vi "get-new-can-frame-by-tag.vi"(8 "error in (no error)":errorcluster, 10 "tag":string, 11 "CANtable in":refnum<class "bAPPdata.lvclass">) -> (0 "error out":errorcluster, 1 "CAN frame":T2 {"payload" format="%x"; "timestamp" format="%<%.7X\n%x>T"; "type" items=["CAN Data"=0, "CAN Remote"=1, "CAN Bus Error"=2, "J1939 Data"=192, "Delay"=224, "Log Trigger"=225, "Start Trigger"=226]; "identifier" format="%x"}, 3 "CANtable out":refnum<class "bAPPdata.lvclass">, 4 "frame.type":T1)   [LabVIEW 2015, in "bAPPdata.lvclass"]
uses:
  bAPPdata.lvclass
  <vilib>/xnet/xnet.llb/XNET Frame CAN.ctl
  <vilib>/xnet/xnet.llb/XNET Frame Type CAN.ctl
  subs/frame.type.ctl
  bAPPdata.lvclass/bAPPdata.ctl
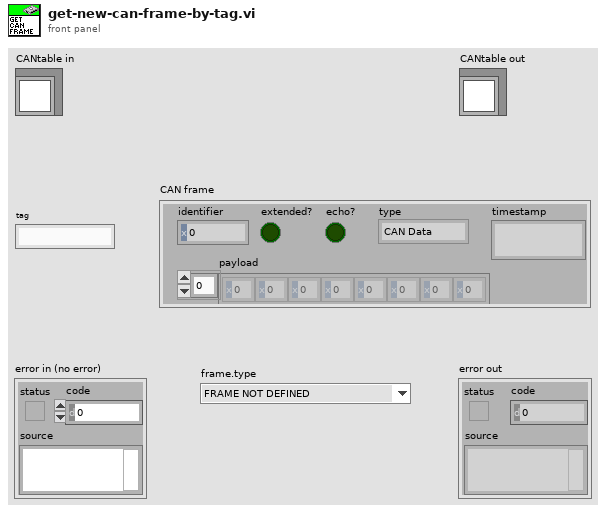
[diagram p1: front panel]
types:
  T1 = typedef "frame.type.ctl" = enum16{"FRAME NOT DEFINED", "DUT OUTPUT FRAME", "DUT INPUT FRAME"}
  T2 = typedef "XNET Frame CAN.ctl" = cluster{"timestamp":timestamp, "payload":u8[], "identifier":u32, "type":T3, "extended?":bool, "echo?":bool}
  T3 = typedef "XNET Frame Type CAN.ctl" = u8
  T4 = typedef "bAPPdata.lvclass/table-data.ctl" = T5[]
  T5 = typedef "bAPPdata.lvclass/table-contents.ctl" = cluster{"id":u32, "tag":string, "frame.type":T1, "last.frame":T2, "tMsgData":T6, "child.tags":string[], "bit-payload":bool[]}
  T6 = typedef "nMsgData.ctl" = cluster{"dwID":u32, "count":u32, "dwCycleTime":dbl, "dwTime":dbl, "new msg":bool}
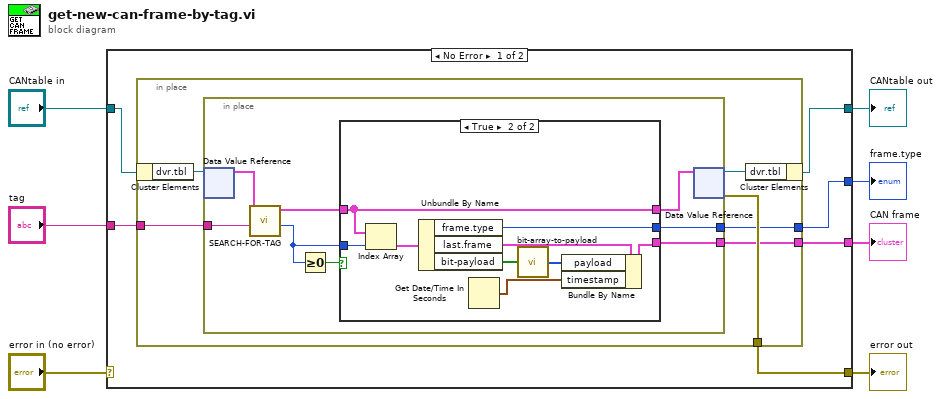
[diagram p0: block diagram]
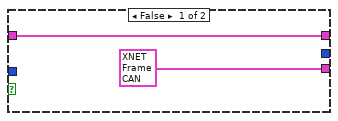
[diagram p2: hidden frame]
diagram:
  n1 = case shown="No Error" "error in (no error)" {
    selector: "error in (no error)" -> [_ w40]
    tunnel: [w8 w40] -> w6
    tunnel: [w12 w39] -> w4
    tunnel: "CANtable in" -> [w13 w39]
    tunnel: "tag" -> [w11 _]
    tunnel: [w10 _] -> w2
    tunnel: [w9 _] -> w1
    frame No Error {
      n2 = in-place {
        in-place-border: w11 -> [w16]
        in-place-border: [w15] -> w10
        in-place-border: [w14] -> w9
        in-place-border: [w19] -> w8
        n3 = in-place-cluster #1(w13) -> ("dvr.tbl"=w18:refnum<data-value>)
        n4 = in-place {
          in-place-border: w16 -> [w26]
          in-place-border: [w22] -> w15
          in-place-border: [w20] -> w14
          n5 = in-place-dvr #2(w18) -> (w27:T4)  [unwired: 1 out]
          n6 = call "SEARCH-FOR-TAG.vi"("tag"=w26, "tbl.list"=w27) -> ("idx"=w21:i32, "tbl.list out"=w24:T5[])  [unwired: 8 in]
          n7 = Greater Or Equal To 0?(x=w21) -> (x >= 0?=w25:bool)
          n8 = case shown="True" w25 {
            tunnel: w24 -> [w29 w38]
            tunnel: [w29 w38] -> w23
            tunnel: [T2 {"timestamp"=timestamp(0 s since 1904-01-01), "payload"=[], "identifier"=0, "type"=0, "extended?"=FALSE, "echo?"=FALSE} ("CAN frame") w34] -> w22
            tunnel: w21 -> [_ w37]
            tunnel: [_ w30] -> w20
            frame False {
            }
            frame True {
              n9 = Index Array(array=w38, index=w37) -> (element=w36:T5)
              n10 = Unbundle By Name(w36) -> ("frame.type"=w30:T1, "last.frame"=w35:T2, "bit-payload"=w32:bool[])
              n11 = Get Date/Time In Seconds() -> (seconds since 1Jan1904=w33:timestamp)
              n12 = call "bit-array-to-payload.vi"("Array"=w32) -> ("payload"=w31:u8[])  [unwired: 4 in]
              n13 = Bundle By Name(cluster=w35, "payload"=w31, "timestamp"=w33) -> (w34:T2)
            }
          }
          n14 = in-place-dvr #2(w23) -> (w17:refnum<data-value>, w19:errorcluster)
        }
        n15 = in-place-cluster #1("dvr.tbl"=w17) -> (w12:refnum<class "bAPPdata.lvclass">)
      }
    }
    frame Error {
    }
  }
  "error out" <- w6
  "CANtable out" <- w4
  "CAN frame" <- w2
  "frame.type" <- w1
